vi "set read out direction.vi"(8 "error in (no error)":errorcluster, 11 "DAQOrcaFlash in":refnum<class "DAQOrcaFlash.lvclass">) -> (0 "error out":errorcluster, 3 "DAQOrcaFlash out":refnum<class "DAQOrcaFlash.lvclass">)   [LabVIEW 2012, in "DAQOrcaFlash.lvclass"]
uses:
  DAQOrcaFlash.lvclass
  DAQOrcaFlash.lvclass/DAQOrcaFlash.ctl
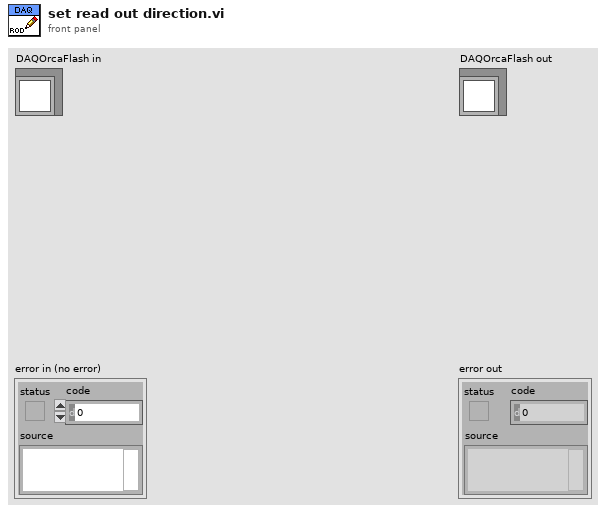
[diagram p1: front panel]
types:
  T1 = typedef "DAQOrcaFlash.lvclass/read out direction.ctl" = sgl
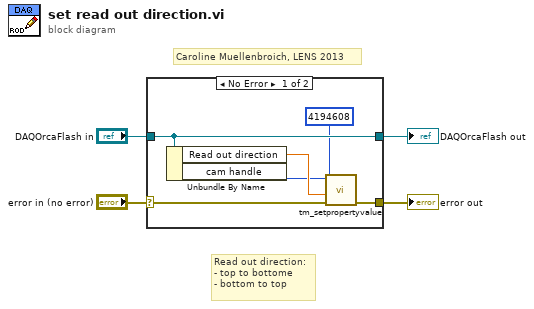
[diagram p0: block diagram]
diagram:
  # "Read out direction:\n- top to bottome\n- bottom to top"
  # "Caroline Muellenbroich, LENS 2013"
  n1 = case shown="No Error" "error in (no error)" {
    selector: "error in (no error)" -> [w10 w12]
    tunnel: [w9 w12] -> w3
    tunnel: [w8 w11] -> w1
    tunnel: "DAQOrcaFlash in" -> [w8 w11]
    frame No Error {
      n2 = Unbundle By Name(w8) -> ("Read out direction"=w6:T1, "cam handle"=w5:u32)
      n3 = call <userlib>:"tm_setpropertyvalue.vi"("error in (no error)"=w10, "Value in"=w6, "Property ID"=u32 4194608, "Handle in"=w5) -> ("error out"=w9:errorcluster)  [unwired: 6 in, 1 out]
    }
    frame Error {
    }
  }
  "error out" <- w3
  "DAQOrcaFlash out" <- w1
